vi "SwissSPAD Live_Get SS2 FPGA Parameters.vi"(6 "Live Mode":bool, 8 "Error In":errorcluster, 10 "Bifile Path":path, 11 "SS2 DAQ Parameters":T1 {"Sync Period" min=0.0 max=4.294967295; "Laser Period" min=0.0 max=4.294967295}) -> (0 "Error Out":errorcluster, 1 "#8-bit Images per Set":u32, 2 "SS2 FPGA DAQ Parameters":u32[](array[numeric]), 3 "SS2 FPGA DAQ Addresses":i32[](array[numeric]), 5 "Discard First Image":bool)   [LabVIEW 2021]
uses:
  SwissSPAD Live_SS2 DAQ Parameters 3.ctl
  SwissSPAD Live_SS2 Gate Definition.ctl
  <vilib>/Utility/error.llb/Error Cluster From Error Code.vi
  <vilib>/ErrorRing/Error Ring.xnode
panel:
  out "Buffer Size (#8-bit Images)":u32
  in  "Current Image Set":i32
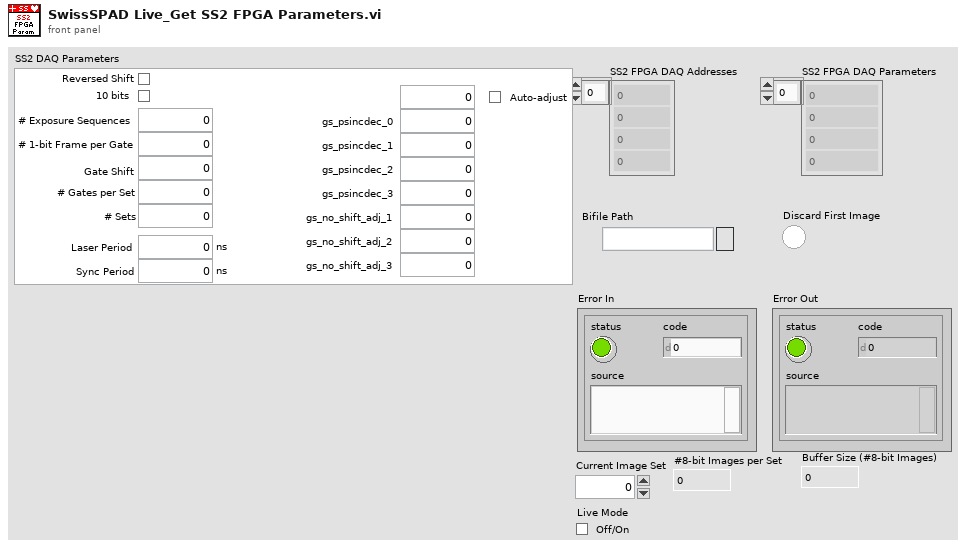
[diagram p1: front panel]
types:
  T1 = typedef "SwissSPAD Live_SS2 DAQ Parameters 3.ctl" = cluster{"10 bits":bool, "# Exposure Sequences":u32, "# 1-bit Frame per Gate":u32, "Gate Shift":u32, "# Gates per Set":u32, "# Sets":u32, "Laser Period":dbl[unit], "Sync Period":dbl[unit], "Gate Offset":u32, "Auto-adjust Gate Offset":bool, "Gate Definition":T2, "Reversed Shift":bool}
  T2 = typedef "SwissSPAD Live_SS2 Gate Definition.ctl" = cluster{"gs_psincdec_0":u32, "gs_psincdec_1":u32, "gs_psincdec_2":u32, "gs_psincdec_3":u32, "gs_no_shift_adj_1":u32, "gs_no_shift_adj_2":u32, "gs_no_shift_adj_3":u32}
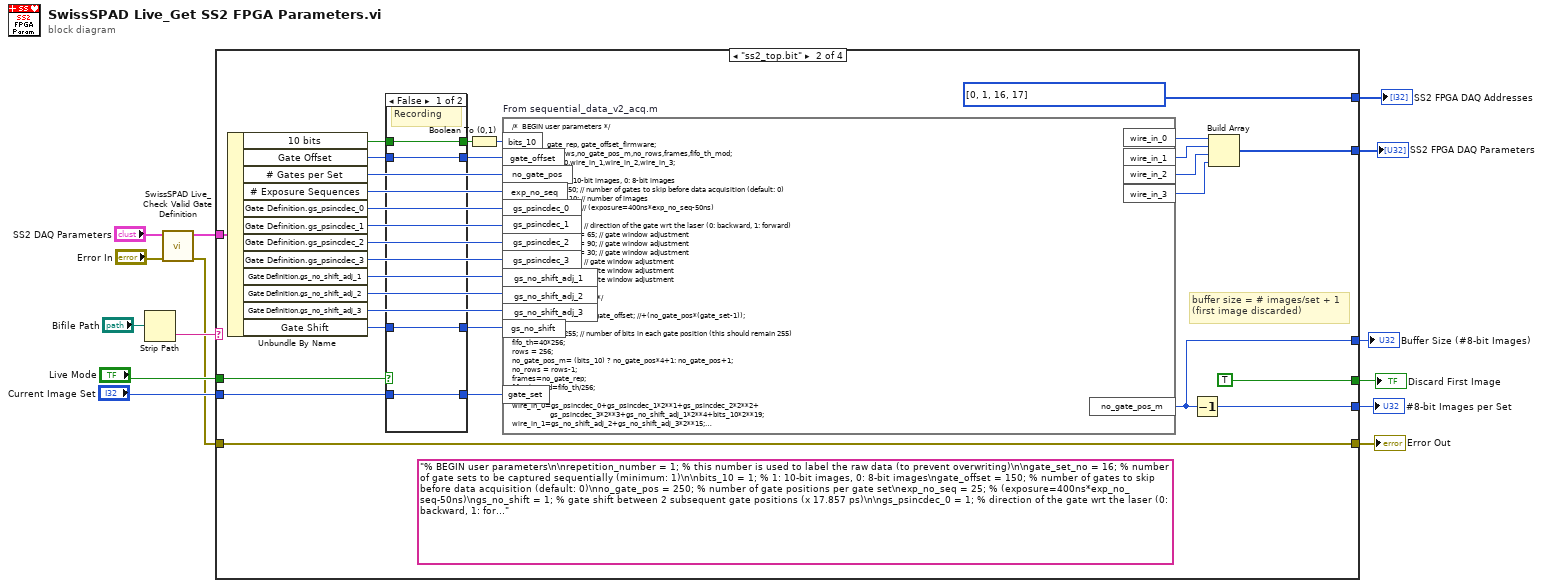
[diagram p0: block diagram]
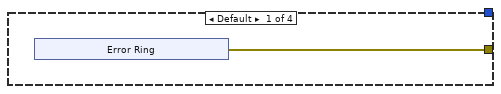
[diagram p2: hidden frame]
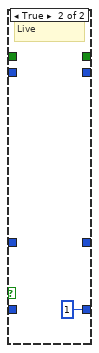
[diagram p3: hidden frame]
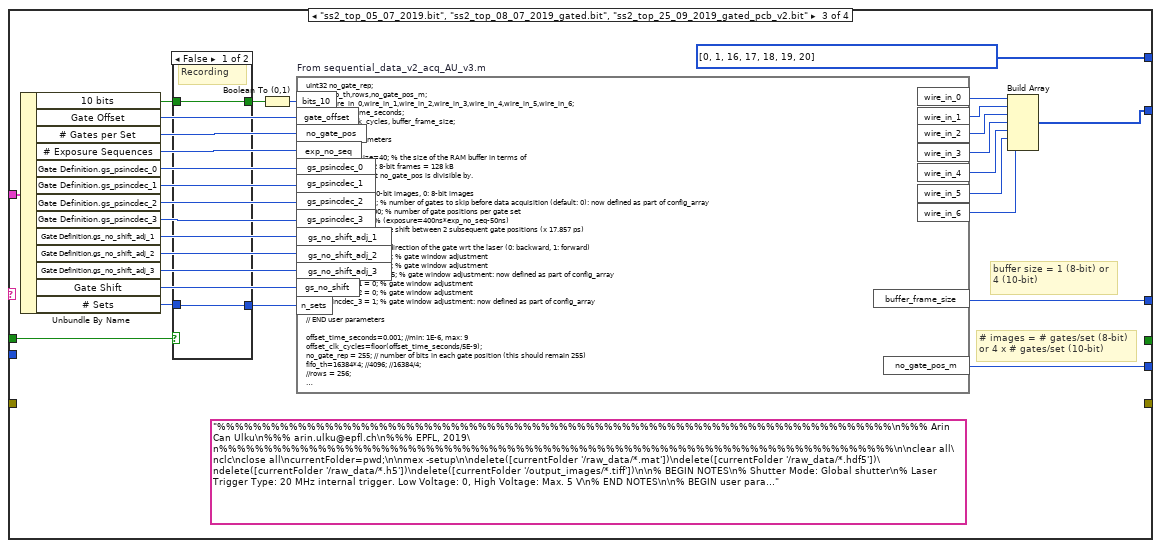
[diagram p4: hidden frame]
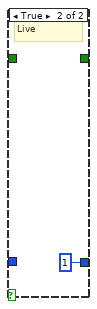
[diagram p5: hidden frame]
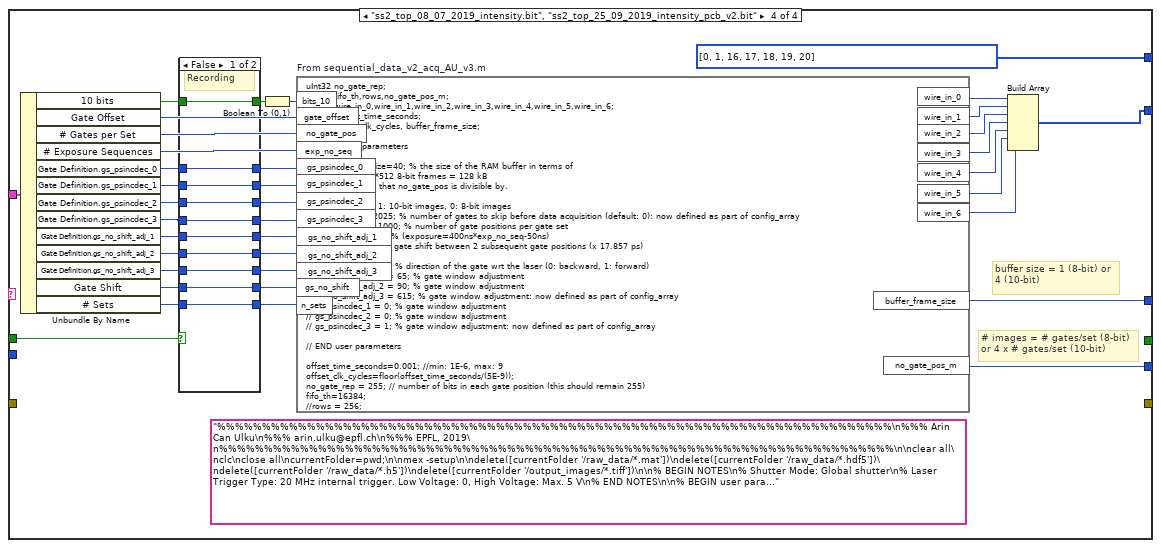
[diagram p6: hidden frame]
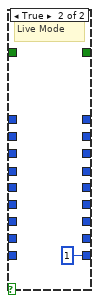
[diagram p7: hidden frame]
diagram:
  n1 = Strip Path(path="Bifile Path") -> (name=w7:string)  [unwired: 1 out]
  n2 = call "SwissSPAD Live_Check Valid Gate Definition.vi"("Error In"="Error In", "SS2 DAQ Parameters in"="SS2 DAQ Parameters") -> ("Error Out"=w4:errorcluster, "SS2 DAQ Parameters out"=w5:T1)  [unwired: 8 in]
  n3 = case shown="\"ss2_top.bit\"" w7 {
    tunnel: [_ w45 w79 w119] -> w14
    tunnel: [_ i32[] [0, 1, 16, 17] ("SS2 FPGA DAQ Addresses") i32[] [0, 1, 16, 17, 18, 19, 20] ("SS2 FPGA DAQ Addresses") i32[] [0, 1, 16, 17, 18, 19, 20] ("SS2 FPGA DAQ Addresses")] -> w13
    tunnel: w5 -> [_ w43 w77 w117]
    tunnel: "Current Image Set" -> [_ w29 _ _]
    tunnel: [_ w24 w69 w105] -> w10
    tunnel: "Live Mode" -> [_ w32 w61 w113]
    tunnel: w4 -> [_ w25 _ _]
    tunnel: [w15 w25 _ _] -> w6
    tunnel: [_ TRUE ("Discard First Image") _ _] -> w2
    tunnel: [_ w22 w56 w88] -> w1
    frame Default {
      n4 = xnode "Error Ring"() -> ("error out"=w15:errorcluster)
    }
    frame "ss2_top.bit" {
      (unwired) "% BEGIN user parameters\n\nrepetition_number = 1; % this number is used to label the raw data (to prevent overwriting)\n\ngate_set_no = 16; % number of gate sets to be captured sequentially (minimum: 1)\n\nbits_10 = 1; % 1: 10-bit images, 0: 8-bit images\ngate_offset = 150; % number of gates to skip before data acquisition (default: 0)\nno_gate_pos = 250; % number of gate positions per gate set\nexp_no_seq = 25; % (exposure=400ns*exp_no_seq-50ns)\ngs_no_shift = 1; % gate shift between 2 subsequent gate positions (x 17.857 ps)\n\ngs_psincdec_0 = 1; % direction of the gate wrt the laser (0: backward, 1: forward)\ngs_no_shift_adj_1 = 65; % gate window adjustment\ngs_no_shift_adj_2 = 90; % gate window adjustment\ngs_no_shift_adj_3 = 85; % gate window adjustment\ngs_psincdec_1 = 0; % gate window adjustment\ngs_psincdec_2 = 0; % gate window adjustment\ngs_psincdec_3 = 0; % gate window adjustment\n\n% END user parameters\n\ndisp('ACQUIRING DATA...')\n\nno_gate_rep = 255; % number of bits in each gate position (this should remain 255)\nfifo_th=40*256;\nrows = 256;\nif bits_10==1\n    no_gate_pos_m=(no_gate_pos*4)+1;\nelse\n    no_gate_pos_m=no_gate_pos+1;\nend\nno_rows = rows-1;\nframes=no_gate_rep;\ngate_set_no_str=int2str(gate_set_no);\nfifo_th_mod=fifo_th/256;\n\nCC=cell(1,gate_set_no);\n\nfor gate_set=1:gate_set_no\n\n    gate_set_str=int2str(gate_set);\n    gate_offset_firmware = gate_offset+(no_gate_pos*(gate_set-1));\n\n    setenv('MW_MINGW64_LOC','C:\\TDM-GCC-64')\n    dev = openFPGA();\n\n    %% ENTER THE BIT FILE DIRECTORY TO THE LINE BELOW %%\n    bitfile = [currentFolder '\\bit_file\\ss2_top.bit'];\n    z_status=configureFPGA(dev, bitfile);\n\n    wire_in_0=gs_psincdec_0+gs_psincdec_1*2^1+gs_psincdec_2*2^2+gs_psincdec_3*2^3+gs_no_shift_adj_1*2^4+bits_10*2^19;\n    setwireinvalue(dev,int32(hex2dec('00')),wire_in_0,wire_in_0)\n    updatewireins(dev)\n    wire_in_1=gs_no_shift_adj_2+gs_no_shift_adj_3*2^15;\n    setwireinvalue(dev,int32(hex2dec('01')),wire_in_1,wire_in_1)\n    updatewireins(dev)\n    wire_in_2=fifo_th_mod+no_gate_pos_m*2^8+gs_no_shift*2^24;\n    setwireinvalue(dev,int32(hex2dec('10')),wire_in_2,wire_in_2)\n    updatewireins(dev)\n    wire_in_3=exp_no_seq+gate_offset_firmware*2^16;\n    setwireinvalue(dev,int32(hex2dec('11')),wire_in_3,wire_in_3)\n    updatewireins(dev)\n\n    % BEGIN SAVE\n\n    activatetriggerin(dev,int32(hex2dec('40')),0)\n    activatetriggerin(dev,int32(hex2dec('40')),1)\n\n    disp(['GATE SET:' gate_set_str '/' gate_set_no_str ' --- ACQUIRING DATA...'])\n    tic\n    CC{gate_set}=readfromblockpipeout(dev,int32(hex2dec('A0')),16*256*4,(512*256)*no_gate_pos_m);\n    toc\n    \n    closeFPGA(dev);"
      # "buffer size = # images/set + 1\n(first image discarded)"
      n5 = Unbundle By Name(w43) -> ("10 bits"=w31:bool, "Gate Offset"=w21:u32, "# Gates per Set"=w41:u32, "# Exposure Sequences"=w40:u32, "Gate Definition.gs_psincdec_0"=w39:u32, "Gate Definition.gs_psincdec_1"=w38:u32, "Gate Definition.gs_psincdec_2"=w37:u32, "Gate Definition.gs_psincdec_3"=w36:u32, "Gate Definition.gs_no_shift_adj_1"=w35:u32, "Gate Definition.gs_no_shift_adj_2"=w34:u32, "Gate Definition.gs_no_shift_adj_3"=w33:u32, "Gate Shift"=w27:u32)
      n6 = case shown="False" w32 {
        tunnel: w31 -> [w53 _]
        tunnel: [w53 _] -> w30
        tunnel: w29 -> [w52 _]
        tunnel: [w52 1 ("Current Image Set")] -> w28
        tunnel: w27 -> [w51 _]
        tunnel: [w51 _] -> w26
        tunnel: w21 -> [w50 _]
        tunnel: [w50 _] -> w20
        frame False {
          # "Recording"
        }
        frame True {
          # "Live"
        }
      }
      n7 = Boolean To (0,1)(Boolean=w30) -> (0, 1=w42:i16)
      n8 = formula code="/*  BEGIN user parameters */\n\nuInt32 no_gate_rep, gate_offset_firmware;\nuInt32 fifo_th,rows,no_gate_pos_m,no_rows,frames,fifo_th_mod;\nuInt32 wire_in_0,wire_in_1,wire_in_2,wire_in_3;\n\n//bits_10 = 0; // 1: 10-bit images, 0: 8-bit images\n//gate_offset = 650; // number of gates to skip before data acquisition (default: 0)\n//no_gate_pos = 10; // number of images\n//exp_no_seq = 100; // (exposure=400ns*exp_no_seq-50ns)\n\n//gs_psincdec_0 = 1; // direction of the gate wrt the laser (0: backward, 1: forward)\n//gs_no_shift_adj_1 = 65; // gate window adjustment\n//gs_no_shift_adj_2 = 90; // gate window adjustment\n//gs_no_shift_adj_3 = 30; // gate window adjustment\n//gs_psincdec_1 = 0; // gate window adjustment\n//gs_psincdec_2 = 0; // gate window adjustment\n//gs_psincdec_3 = 0; // gate window adjustment\n\n/*  END user parameters */\n\ngate_offset_firmware = gate_offset; //+(no_gate_pos*(gate_set-1));\n\nno_gate_rep = 255; // number of bits in each gate position (this should remain 255)\nfifo_th=40*256;\nrows = 256;\nno_gate_pos_m= (bits_10) ? no_gate_pos*4+1: no_gate_pos+1;\nno_rows = rows-1;\nframes=no_gate_rep;\nfifo_th_mod=fifo_th/256;\n\nwire_in_0=gs_psincdec_0+gs_psincdec_1*2**1+gs_psincdec_2*2**2+\n                   gs_psincdec_3*2**3+gs_no_shift_adj_1*2**4+bits_10*2**19;\nwire_in_1=gs_no_shift_adj_2+gs_no_shift_adj_3*2**15;\nwire_in_2=fifo_th_mod+no_gate_pos_m*2**8+gs_no_shift*2**24;\nwire_in_3=exp_no_seq+gate_offset_firmware*2**16;" "From sequential_data_v2_acq.m"("bits_10"=w42, "gate_offset"=w20, "no_gate_pos"=w41, "exp_no_seq"=w40, "gs_psincdec_0"=w39, "gs_psincdec_1"=w38, "gs_psincdec_2"=w37, "gs_psincdec_3"=w36, "gs_no_shift_adj_1"=w35, "gs_no_shift_adj_2"=w34, "gs_no_shift_adj_3"=w33, "gate_set"=w28, "gs_no_shift"=w26) -> ("wire_in_1"=w48:u32, "wire_in_0"=w49:u32, "wire_in_2"=w47:u32, "wire_in_3"=w46:u32, "no_gate_pos_m"=w22:u32)
      n9 = Decrement(x=w22) -> (x-1=w24:u32)
      n10 = Build Array(w49, w48, w47, w46) -> (w45:u32[])
    }
    frame "ss2_top_05_07_2019.bit", "ss2_top_08_07_2019_gated.bit", "ss2_top_25_09_2019_gated_pcb_v2.bit" {
      (unwired) "%%%%%%%%%%%%%%%%%%%%%%%%%%%%%%%%%%%%%%%%%%%%%%%%%%%%%%%%%%%%%%%%%%%%%%%%%%%\n%%% Arin Can Ulku\n%%% arin.ulku@epfl.ch\n%%% EPFL, 2019\n%%%%%%%%%%%%%%%%%%%%%%%%%%%%%%%%%%%%%%%%%%%%%%%%%%%%%%%%%%%%%%%%%%%%%%%%%%%\n\nclear all\nclc\nclose all\ncurrentFolder=pwd;\n\nmex -setup\n\ndelete([currentFolder '/raw_data/*.mat'])\ndelete([currentFolder '/raw_data/*.hdf5'])\ndelete([currentFolder '/raw_data/*.h5'])\ndelete([currentFolder '/output_images/*.tiff'])\n\n% BEGIN NOTES\n% Shutter Mode: Global shutter\n% Laser Trigger Type: 20 MHz internal trigger. Low Voltage: 0, High Voltage: Max. 5 V\n% END NOTES\n\n% BEGIN user parameters\n\n%%%%%%%%%%%%%%%%%%%%%%%%%%%%%%%%%%%%%%%%%%%%%%%%%%%%%\n% Added by XM for hdf5 saving and automation purposes\n\nfile_root_name = 'DCR study'; % root file name\nrepetition_number = 1;                 % number of repetitions per config\nrepetition_number_str = int2str(repetition_number);\nconfig_choice = [3];                 % define which config(s) to use\n% For all config, use [1 2 3 4 5 6 7]\n% For a single config, e.g. 3, use [3]\nconfig_number = length(config_choice);\n\n% Don't modify the array below unless you know what you are doing...\nconfig_array = struct('gate_offset', {2690,2640,2570,2430,2300,2170,2025},...\n    'gs_no_shift_adj_3',{85,30,55,195,335,475,615},...\n    'gs_psincdec_3',{0,0,1,1,1,1,1},...\n    'gate_width_ns',{10.8,11.7,13.1,15.5,17.9,20.3,22.8});\n% offset array for Arin's series: {2690,2640,2570,2430,2300,2170,2025}\nfile_version = 'SS2 0.1';               % do not modify\nsoftware_name = 'sequential_data_v2_acq.m'; % do not modify\nsoftware_version = '64-bit';            % do not modify\nfirmware_name = 'ss2_top_05_07_2019.bit';          % do not modify\nfirmware_version = '07-05-2019';        % modify when firmware has been updated\nsample_description = 'DCR Study as a function of integration time'; % user-defined\nauthor = 'X. Michalet';                 % user-defined\nlaser_f_MHz = 20;                       % do not modify\npixel_x = 512;                          % do not modify\npixel_y = 256;                          % do not modify\ngate_step_ps = 17.857;                  % do not modify, might change if firmware changes\n\n% end XM additions\n%%%%%%%%%%%%%%%%%%%%%%%%%%%%%%%%%%%%%%\n\nbuffer_frame_size=40; % the size of the RAM buffer in terms of equivalent 256*512 frames\n% choose a value that no_gate_pos is divisible by.\n\nbits_10 = 0; % 1: 10-bit images, 0: 8-bit images\n%gate_offset = 2025; % number of gates to skip before data acquisition (default: 0): now defined as part of config_array\nno_gate_pos = 1000; % number of gate positions per gate set\nexp_no_seq = 25; % (exposure=400ns*exp_no_seq-50ns)\ngs_no_shift = 1; % gate shift between 2 subsequent gate positions (x 17.857 ps)\n\ngs_psincdec_0 = 1; % direction of the gate wrt the laser (0: backward, 1: forward)\ngs_no_shift_adj_1 = 65; % gate window adjustment\ngs_no_shift_adj_2 = 90; % gate window adjustment\n%gs_no_shift_adj_3 = 615; % gate window adjustment: now defined as part of config_array\ngs_psincdec_1 = 0; % gate window adjustment\ngs_psincdec_2 = 0; % gate window adjustment\n%gs_psincdec_3 = 1; % gate window adjustment: now defined as part of config_array\n\n% END user parameters\n\ngate_set_no = 1; % number of gate sets to be captured sequentially (minimum: 1)\noffset_time_seconds=0.001; %% min: 1E-6, max: 9\noffset_clk_cycles=floor(offset_time_seconds/(5E-9));\nno_gate_rep = 255; % number of bits in each gate position (this should remain 255)\nfifo_th=16384/4;\nrows = 256;\nif bits_10==1\n    no_gate_pos_m=(no_gate_pos*4);\nelse\n    no_gate_pos_m=no_gate_pos;\nend\nno_rows = rows-1;\nframes=no_gate_rep;\n\nsetenv('MW_MINGW64_LOC','C:\\TDM-GCC-64')\ndev = openFPGA();\nbitfile = [currentFolder '\\bit_file\\ss2_top_08_07_2019_intensity.bit'];\nz_status=configureFPGA(dev, bitfile);\n\nfor j=1:config_number\n    config = config_choice(j);\n    gate_offset = config_array(config).gate_offset;\n    gs_no_shift_adj_3 = config_array(config).gs_no_shift_adj_3;\n    gs_psincdec_3 = config_array(config).gs_psincdec_3;\n    gate_width_ns = config_array(config).gate_width_ns;\n    config_number_str = [' (config ' int2str(config) ')'];\n    file_name = [file_root_name config_number_str];\n    \n    %%%%%%%%%%%%%%%%%%%%%%%%%%%%%%%%%%%%%%\n    % Added by XM for hdf5 saving purposes\n\n    hdf5write([currentFolder '\\raw_data\\' file_name '.hdf5'],'/SS2_file_version',file_version);\n    hdf5write([currentFolder '\\raw_data\\' file_name '.hdf5'],'/daq_parameters/pixel_x',pixel_x,'WriteMode', 'append');\n    hdf5write([currentFolder '\\raw_data\\' file_name '.hdf5'],'/daq_parameters/pixel_y',pixel_y,'WriteMode', 'append');\n    hdf5write([currentFolder '\\raw_data\\' file_name '.hdf5'],'/daq_parameters/gate_set_no',gate_set_no,'WriteMode', 'append');\n    hdf5write([currentFolder '\\raw_data\\' file_name '.hdf5'],'/daq_parameters/bits_10',bits_10,'WriteMode', 'append');\n    hdf5write([currentFolder '\\raw_data\\' file_name '.hdf5'],'/daq_parameters/gate_offset',gate_offset,'WriteMode', 'append');\n    hdf5write([currentFolder '\\raw_data\\' file_name '.hdf5'],'/daq_parameters/no_gate_pos',no_gate_pos,'WriteMode', 'append');\n    hdf5write([currentFolder '\\raw_data\\' file_name '.hdf5'],'/daq_parameters/exp_no_seq',exp_no_seq,'WriteMode', 'append');\n    hdf5write([currentFolder '\\raw_data\\' file_name '.hdf5'],'/daq_parameters/gs_no_shift',gs_no_shift,'WriteMode', 'append');\n    hdf5write([currentFolder '\\raw_data\\' file_name '.hdf5'],'/daq_parameters/gs_psincdec_0',gs_psincdec_0,'WriteMode', 'append');\n    hdf5write([currentFolder '\\raw_data\\' file_name '.hdf5'],'/daq_parameters/gs_no_shift_adj_1',gs_no_shift_adj_1,'WriteMode', 'append');\n    hdf5write([currentFolder '\\raw_data\\' file_name '.hdf5'],'/daq_parameters/gs_no_shift_adj_2',gs_no_shift_adj_2,'WriteMode', 'append');\n    hdf5write([currentFolder '\\raw_data\\' file_name '.hdf5'],'/daq_parameters/gs_no_shift_adj_3',gs_no_shift_adj_3,'WriteMode', 'append');\n    hdf5write([currentFolder '\\raw_data\\' file_name '.hdf5'],'/daq_parameters/gs_psincdec_1',gs_psincdec_1,'WriteMode', 'append');\n    hdf5write([currentFolder '\\raw_data\\' file_name '.hdf5'],'/daq_parameters/gs_psincdec_2',gs_psincdec_2,'WriteMode', 'append');\n    hdf5write([currentFolder '\\raw_data\\' file_name '.hdf5'],'/daq_parameters/gs_psincdec_3',gs_psincdec_3,'WriteMode', 'append');\n    hdf5write([currentFolder '\\raw_data\\' file_name '.hdf5'],'/daq_parameters/gate_step_ps',gate_step_ps,'WriteMode', 'append');\n    hdf5write([currentFolder '\\raw_data\\' file_name '.hdf5'],'/daq_parameters/gate_width_ns',gate_width_ns,'WriteMode', 'append');\n    hdf5write([currentFolder '\\raw_data\\' file_name '.hdf5'],'/daq_parameters/shutter_mode','global shutter','WriteMode', 'append');\n    hdf5write([currentFolder '\\raw_data\\' file_name '.hdf5'],'/daq_parameters/laser_f_MHz',laser_f_MHz,'WriteMode', 'append');\n\n    hdf5write([currentFolder '\\raw_data\\' file_name '.hdf5'],'/data_information/description',[sample_description config_number_str],'WriteMode', 'append');\n    hdf5write([currentFolder '\\raw_data\\' file_name '.hdf5'],'/data_information/author',author,'WriteMode', 'append');\n    hdf5write([currentFolder '\\raw_data\\' file_name '.hdf5'],'/data_information/software_name',software_name,'WriteMode', 'append');\n    hdf5write([currentFolder '\\raw_data\\' file_name '.hdf5'],'/data_information/software_version',software_version,'WriteMode', 'append');\n    hdf5write([currentFolder '\\raw_data\\' file_name '.hdf5'],'/data_information/firmware_name',firmware_name,'WriteMode', 'append');\n    hdf5write([currentFolder '\\raw_data\\' file_name '.hdf5'],'/data_information/firmware_version',firmware_version,'WriteMode', 'append');\n\n\n    for i=1:repetition_number\n%         exp_no_seq = 10*i;\n        repetition_number_str = [' exp = ' int2str(exp_no_seq)];       \n\n        wire_in_0=gs_psincdec_0+gs_psincdec_1*2^1+gs_psincdec_2*2^2+gs_psincdec_3*2^3+gs_no_shift_adj_1*2^4+bits_10*2^19;\n        setwireinvalue(dev,int32(hex2dec('00')),wire_in_0,wire_in_0)\n        updatewireins(dev)\n        wire_in_1=gs_no_shift_adj_2+gs_no_shift_adj_3*2^15;\n        setwireinvalue(dev,int32(hex2dec('01')),wire_in_1,wire_in_1)\n        updatewireins(dev)\n        wire_in_2=no_gate_pos_m*2^8;\n        setwireinvalue(dev,int32(hex2dec('10')),wire_in_2,wire_in_2)\n        updatewireins(dev)\n        wire_in_3=exp_no_seq+gate_offset*2^16;\n        setwireinvalue(dev,int32(hex2dec('11')),wire_in_3,wire_in_3)\n        updatewireins(dev)\n        wire_in_4=gs_no_shift;\n        setwireinvalue(dev,int32(hex2dec('12')),wire_in_4,wire_in_4)\n        updatewireins(dev)\n        wire_in_5=fifo_th;\n        setwireinvalue(dev,int32(hex2dec('13')),wire_in_5,wire_in_5)\n        updatewireins(dev)\n        wire_in_6=offset_clk_cycles;\n        setwireinvalue(dev,int32(hex2dec('14')),wire_in_6,wire_in_6)\n        updatewireins(dev)\n\n        % BEGIN SAVE\n\n        rep_no=fix(no_gate_pos_m/buffer_frame_size);\n        [daq_time]=ss2_daq_hdf5_v3(file_name,rep_no,dev,int32(hex2dec('A0')),16384,(512*256)*buffer_frame_size);\n    \n        %%%%%%%%%%%%%%%%%%%%%%%%%%%%%%%%%%%%%%\n        % Added by XM for hdf5 saving purposes\n\n        disp(['Elapsed DAQ time: ' num2str(daq_time) ' sec']);\n\n        % end XM additions\n        %%%%%%%%%%%%%%%%%%%%%%%%%%%%%%%%%%%%%%\n\n%         updatewireouts(dev);\n%         fsm_state = dec2hex(getwireoutvalue(dev,int32(hex2dec('20'))));    \n        updatewireouts(dev);\n        fsm_state_2 = dec2hex(getwireoutvalue(dev,int32(hex2dec('21'))));\n\n        beep\n \n        disp([10 'ACQUISITION COMPLETED. YOU CAN TURN OFF THE LASER NOW.' 10])\n%         fsm_state_int=str2double(fsm_state_2);\n%         if fsm_state_int==2\n%             disp(['USB DATA TRANSFER SUCCESSFUL!' 10])\n%         else\n%             disp(['USB DATA TRANSFER FAILED!' 10])\n%         end\n        \n%         file_number_str=int2str(i);\n%         disp(['SAVING HDF5 RAW DATA... File ' file_number_str ' of ' repetition_number_str config_number_str 10])\n\n    end\nend\n\ncloseFPGA(dev);\n\nhdf5write([currentFolder '\\raw_data\\' file_name '.hdf5'],'/daq_time_s',daq_time,'WriteMode', 'append');\n\n% end XM additions\n%%%%%%%%%%%%%%%%%%%%%%%%%%%%%%%%%%%%%%\n    \n%% \n\n%%%%%%%%%%%%%%%%%%%%%%%%%%%%%%%%%%%%%%\n% Added by AU for testing purposes\n\n% disp([10 'SAVING .MAT RAW DATA...' 10])\n% \n% tic\n% \n% save([currentFolder '\\raw_data\\raw_data_1.mat'],'SS2_DATA', '-v7.3');\n% \n% toc\n\n% end AU additions\n%%%%%%%%%%%%%%%%%%%%%%%%%%%%%%%%%%%%%%\n\ndisp([10 'DONE.'])\n\n%disp('SAVING MATLAB RAW DATA...')\n\n%tic\n%save([currentFolder '\\raw_data\\' file_name '_' file_number_str '.mat'],'CC');\n%toc\n\nbeep"
      # "# images = # gates/set (8-bit)\nor 4 x # gates/set (10-bit)"
      # "buffer size = 1 (8-bit) or 4 (10-bit)"
      n11 = Unbundle By Name(w77) -> ("10 bits"=w60:bool, "Gate Offset"=w55:u32, "# Gates per Set"=w75:u32, "# Exposure Sequences"=w74:u32, "Gate Definition.gs_psincdec_0"=w68:u32, "Gate Definition.gs_psincdec_1"=w67:u32, "Gate Definition.gs_psincdec_2"=w66:u32, "Gate Definition.gs_psincdec_3"=w65:u32, "Gate Definition.gs_no_shift_adj_1"=w64:u32, "Gate Definition.gs_no_shift_adj_2"=w63:u32, "Gate Definition.gs_no_shift_adj_3"=w62:u32, "Gate Shift"=w73:u32, "# Sets"=w58:u32)
      n12 = case shown="False" w61 {
        tunnel: w60 -> [w85 _]
        tunnel: [w85 _] -> w59
        tunnel: w58 -> [w84 _]
        tunnel: [w84 u32 1 ("# Sets")] -> w57
        frame False {
          # "Recording"
        }
        frame True {
          # "Live"
        }
      }
      n13 = Boolean To (0,1)(Boolean=w59) -> (0, 1=w76:i16)
      n14 = formula code="uInt32 no_gate_rep;\nuInt32 fifo_th,rows,no_gate_pos_m;\nuInt32 wire_in_0,wire_in_1,wire_in_2,wire_in_3,wire_in_4,wire_in_5,wire_in_6;\nfloat64 offset_time_seconds;\nuInt32 offset_clk_cycles, buffer_frame_size;\n\n// BEGIN user parameters\n\n// buffer_frame_size=40; % the size of the RAM buffer in terms of \n// equivalent 256*512 8-bit frames = 128 kB\n// choose a value that no_gate_pos is divisible by.\n\n// bits_10 = 0; % 1: 10-bit images, 0: 8-bit images\n// gate_offset = 2025; % number of gates to skip before data acquisition (default: 0): now defined as part of config_array\n// no_gate_pos = 1000; % number of gate positions per gate set\n// exp_no_seq = 25; % (exposure=400ns*exp_no_seq-50ns)\n// gs_no_shift = 1; % gate shift between 2 subsequent gate positions (x 17.857 ps)\n\n// gs_psincdec_0 = 1; % direction of the gate wrt the laser (0: backward, 1: forward)\n// gs_no_shift_adj_1 = 65; % gate window adjustment\n// gs_no_shift_adj_2 = 90; % gate window adjustment\n// gs_no_shift_adj_3 = 615; % gate window adjustment: now defined as part of config_array\n// gs_psincdec_1 = 0; % gate window adjustment\n// gs_psincdec_2 = 0; % gate window adjustment\n// gs_psincdec_3 = 1; % gate window adjustment: now defined as part of config_array\n\n// END user parameters\n\noffset_time_seconds=0.001; //min: 1E-6, max: 9\noffset_clk_cycles=floor(offset_time_seconds/5E-9);\nno_gate_rep = 255; // number of bits in each gate position (this should remain 255)\nfifo_th=16384*4; //4096; //16384/4;\n//rows = 256;\n\n no_gate_pos_m = (bits_10 ==1) ? no_gate_pos*4 : no_gate_pos;\nbuffer_frame_size = (bits_10 ==1) ? 4 : 1;\n//= no_gate_pos_m; // e.g. bits_10 = 1, no_gate_pos = 100 >> buffer = 50 MB\n//no_gate_pos_m *= n_sets; \n\n//no_rows = rows-1;\n//frames=no_gate_rep;\n\nwire_in_0=gs_psincdec_0+gs_psincdec_1*2**1+gs_psincdec_2*2**2+gs_psincdec_3*2**3+gs_no_shift_adj_1*2**4+bits_10*2**19;\nwire_in_1=gs_no_shift_adj_2+gs_no_shift_adj_3*2**15;\nwire_in_2=no_gate_pos_m*2**8;\nwire_in_3=exp_no_seq+gate_offset*2**16;\nwire_in_4=gs_no_shift;\nwire_in_5=fifo_th;\nwire_in_6=offset_clk_cycles;" "From sequential_data_v2_acq_AU_v3.m"("bits_10"=w76, "gate_offset"=w55, "no_gate_pos"=w75, "exp_no_seq"=w74, "gs_psincdec_0"=w68, "gs_psincdec_1"=w67, "gs_psincdec_2"=w66, "gs_psincdec_3"=w65, "gs_no_shift_adj_1"=w64, "gs_no_shift_adj_2"=w63, "gs_no_shift_adj_3"=w62, "gs_no_shift"=w73, "n_sets"=w57) -> ("wire_in_1"=w82:u32, "wire_in_0"=w83:u32, "wire_in_2"=w81:u32, "wire_in_3"=w80:u32, "no_gate_pos_m"=w69:u32, "wire_in_4"=w72:u32, "wire_in_5"=w71:u32, "wire_in_6"=w70:u32, "buffer_frame_size"=w56:u32)
      n15 = Build Array(w83, w82, w81, w80, w72, w71, w70) -> (w79:u32[])
    }
    frame "ss2_top_08_07_2019_intensity.bit", "ss2_top_25_09_2019_intensity_pcb_v2.bit" {
      (unwired) "%%%%%%%%%%%%%%%%%%%%%%%%%%%%%%%%%%%%%%%%%%%%%%%%%%%%%%%%%%%%%%%%%%%%%%%%%%%\n%%% Arin Can Ulku\n%%% arin.ulku@epfl.ch\n%%% EPFL, 2019\n%%%%%%%%%%%%%%%%%%%%%%%%%%%%%%%%%%%%%%%%%%%%%%%%%%%%%%%%%%%%%%%%%%%%%%%%%%%\n\nclear all\nclc\nclose all\ncurrentFolder=pwd;\n\nmex -setup\n\ndelete([currentFolder '/raw_data/*.mat'])\ndelete([currentFolder '/raw_data/*.hdf5'])\ndelete([currentFolder '/raw_data/*.h5'])\ndelete([currentFolder '/output_images/*.tiff'])\n\n% BEGIN NOTES\n% Shutter Mode: Global shutter\n% Laser Trigger Type: 20 MHz internal trigger. Low Voltage: 0, High Voltage: Max. 5 V\n% END NOTES\n\n% BEGIN user parameters\n\n%%%%%%%%%%%%%%%%%%%%%%%%%%%%%%%%%%%%%%%%%%%%%%%%%%%%%\n% Added by XM for hdf5 saving and automation purposes\n\nfile_root_name = 'DCR study'; % root file name\nrepetition_number = 1;                 % number of repetitions per config\nrepetition_number_str = int2str(repetition_number);\nconfig_choice = [3];                 % define which config(s) to use\n% For all config, use [1 2 3 4 5 6 7]\n% For a single config, e.g. 3, use [3]\nconfig_number = length(config_choice);\n\n% Don't modify the array below unless you know what you are doing...\nconfig_array = struct('gate_offset', {2690,2640,2570,2430,2300,2170,2025},...\n    'gs_no_shift_adj_3',{85,30,55,195,335,475,615},...\n    'gs_psincdec_3',{0,0,1,1,1,1,1},...\n    'gate_width_ns',{10.8,11.7,13.1,15.5,17.9,20.3,22.8});\n% offset array for Arin's series: {2690,2640,2570,2430,2300,2170,2025}\nfile_version = 'SS2 0.1';               % do not modify\nsoftware_name = 'sequential_data_v2_acq.m'; % do not modify\nsoftware_version = '64-bit';            % do not modify\nfirmware_name = 'ss2_top_05_07_2019.bit';          % do not modify\nfirmware_version = '07-05-2019';        % modify when firmware has been updated\nsample_description = 'DCR Study as a function of integration time'; % user-defined\nauthor = 'X. Michalet';                 % user-defined\nlaser_f_MHz = 20;                       % do not modify\npixel_x = 512;                          % do not modify\npixel_y = 256;                          % do not modify\ngate_step_ps = 17.857;                  % do not modify, might change if firmware changes\n\n% end XM additions\n%%%%%%%%%%%%%%%%%%%%%%%%%%%%%%%%%%%%%%\n\nbuffer_frame_size=40; % the size of the RAM buffer in terms of equivalent 256*512 frames\n% choose a value that no_gate_pos is divisible by.\n\nbits_10 = 0; % 1: 10-bit images, 0: 8-bit images\n%gate_offset = 2025; % number of gates to skip before data acquisition (default: 0): now defined as part of config_array\nno_gate_pos = 1000; % number of gate positions per gate set\nexp_no_seq = 25; % (exposure=400ns*exp_no_seq-50ns)\ngs_no_shift = 1; % gate shift between 2 subsequent gate positions (x 17.857 ps)\n\ngs_psincdec_0 = 1; % direction of the gate wrt the laser (0: backward, 1: forward)\ngs_no_shift_adj_1 = 65; % gate window adjustment\ngs_no_shift_adj_2 = 90; % gate window adjustment\n%gs_no_shift_adj_3 = 615; % gate window adjustment: now defined as part of config_array\ngs_psincdec_1 = 0; % gate window adjustment\ngs_psincdec_2 = 0; % gate window adjustment\n%gs_psincdec_3 = 1; % gate window adjustment: now defined as part of config_array\n\n% END user parameters\n\ngate_set_no = 1; % number of gate sets to be captured sequentially (minimum: 1)\noffset_time_seconds=0.001; %% min: 1E-6, max: 9\noffset_clk_cycles=floor(offset_time_seconds/(5E-9));\nno_gate_rep = 255; % number of bits in each gate position (this should remain 255)\nfifo_th=16384/4;\nrows = 256;\nif bits_10==1\n    no_gate_pos_m=(no_gate_pos*4);\nelse\n    no_gate_pos_m=no_gate_pos;\nend\nno_rows = rows-1;\nframes=no_gate_rep;\n\nsetenv('MW_MINGW64_LOC','C:\\TDM-GCC-64')\ndev = openFPGA();\nbitfile = [currentFolder '\\bit_file\\ss2_top_08_07_2019_intensity.bit'];\nz_status=configureFPGA(dev, bitfile);\n\nfor j=1:config_number\n    config = config_choice(j);\n    gate_offset = config_array(config).gate_offset;\n    gs_no_shift_adj_3 = config_array(config).gs_no_shift_adj_3;\n    gs_psincdec_3 = config_array(config).gs_psincdec_3;\n    gate_width_ns = config_array(config).gate_width_ns;\n    config_number_str = [' (config ' int2str(config) ')'];\n    file_name = [file_root_name config_number_str];\n    \n    %%%%%%%%%%%%%%%%%%%%%%%%%%%%%%%%%%%%%%\n    % Added by XM for hdf5 saving purposes\n\n    hdf5write([currentFolder '\\raw_data\\' file_name '.hdf5'],'/SS2_file_version',file_version);\n    hdf5write([currentFolder '\\raw_data\\' file_name '.hdf5'],'/daq_parameters/pixel_x',pixel_x,'WriteMode', 'append');\n    hdf5write([currentFolder '\\raw_data\\' file_name '.hdf5'],'/daq_parameters/pixel_y',pixel_y,'WriteMode', 'append');\n    hdf5write([currentFolder '\\raw_data\\' file_name '.hdf5'],'/daq_parameters/gate_set_no',gate_set_no,'WriteMode', 'append');\n    hdf5write([currentFolder '\\raw_data\\' file_name '.hdf5'],'/daq_parameters/bits_10',bits_10,'WriteMode', 'append');\n    hdf5write([currentFolder '\\raw_data\\' file_name '.hdf5'],'/daq_parameters/gate_offset',gate_offset,'WriteMode', 'append');\n    hdf5write([currentFolder '\\raw_data\\' file_name '.hdf5'],'/daq_parameters/no_gate_pos',no_gate_pos,'WriteMode', 'append');\n    hdf5write([currentFolder '\\raw_data\\' file_name '.hdf5'],'/daq_parameters/exp_no_seq',exp_no_seq,'WriteMode', 'append');\n    hdf5write([currentFolder '\\raw_data\\' file_name '.hdf5'],'/daq_parameters/gs_no_shift',gs_no_shift,'WriteMode', 'append');\n    hdf5write([currentFolder '\\raw_data\\' file_name '.hdf5'],'/daq_parameters/gs_psincdec_0',gs_psincdec_0,'WriteMode', 'append');\n    hdf5write([currentFolder '\\raw_data\\' file_name '.hdf5'],'/daq_parameters/gs_no_shift_adj_1',gs_no_shift_adj_1,'WriteMode', 'append');\n    hdf5write([currentFolder '\\raw_data\\' file_name '.hdf5'],'/daq_parameters/gs_no_shift_adj_2',gs_no_shift_adj_2,'WriteMode', 'append');\n    hdf5write([currentFolder '\\raw_data\\' file_name '.hdf5'],'/daq_parameters/gs_no_shift_adj_3',gs_no_shift_adj_3,'WriteMode', 'append');\n    hdf5write([currentFolder '\\raw_data\\' file_name '.hdf5'],'/daq_parameters/gs_psincdec_1',gs_psincdec_1,'WriteMode', 'append');\n    hdf5write([currentFolder '\\raw_data\\' file_name '.hdf5'],'/daq_parameters/gs_psincdec_2',gs_psincdec_2,'WriteMode', 'append');\n    hdf5write([currentFolder '\\raw_data\\' file_name '.hdf5'],'/daq_parameters/gs_psincdec_3',gs_psincdec_3,'WriteMode', 'append');\n    hdf5write([currentFolder '\\raw_data\\' file_name '.hdf5'],'/daq_parameters/gate_step_ps',gate_step_ps,'WriteMode', 'append');\n    hdf5write([currentFolder '\\raw_data\\' file_name '.hdf5'],'/daq_parameters/gate_width_ns',gate_width_ns,'WriteMode', 'append');\n    hdf5write([currentFolder '\\raw_data\\' file_name '.hdf5'],'/daq_parameters/shutter_mode','global shutter','WriteMode', 'append');\n    hdf5write([currentFolder '\\raw_data\\' file_name '.hdf5'],'/daq_parameters/laser_f_MHz',laser_f_MHz,'WriteMode', 'append');\n\n    hdf5write([currentFolder '\\raw_data\\' file_name '.hdf5'],'/data_information/description',[sample_description config_number_str],'WriteMode', 'append');\n    hdf5write([currentFolder '\\raw_data\\' file_name '.hdf5'],'/data_information/author',author,'WriteMode', 'append');\n    hdf5write([currentFolder '\\raw_data\\' file_name '.hdf5'],'/data_information/software_name',software_name,'WriteMode', 'append');\n    hdf5write([currentFolder '\\raw_data\\' file_name '.hdf5'],'/data_information/software_version',software_version,'WriteMode', 'append');\n    hdf5write([currentFolder '\\raw_data\\' file_name '.hdf5'],'/data_information/firmware_name',firmware_name,'WriteMode', 'append');\n    hdf5write([currentFolder '\\raw_data\\' file_name '.hdf5'],'/data_information/firmware_version',firmware_version,'WriteMode', 'append');\n\n\n    for i=1:repetition_number\n%         exp_no_seq = 10*i;\n        repetition_number_str = [' exp = ' int2str(exp_no_seq)];       \n\n        wire_in_0=gs_psincdec_0+gs_psincdec_1*2^1+gs_psincdec_2*2^2+gs_psincdec_3*2^3+gs_no_shift_adj_1*2^4+bits_10*2^19;\n        setwireinvalue(dev,int32(hex2dec('00')),wire_in_0,wire_in_0)\n        updatewireins(dev)\n        wire_in_1=gs_no_shift_adj_2+gs_no_shift_adj_3*2^15;\n        setwireinvalue(dev,int32(hex2dec('01')),wire_in_1,wire_in_1)\n        updatewireins(dev)\n        wire_in_2=no_gate_pos_m*2^8;\n        setwireinvalue(dev,int32(hex2dec('10')),wire_in_2,wire_in_2)\n        updatewireins(dev)\n        wire_in_3=exp_no_seq+gate_offset*2^16;\n        setwireinvalue(dev,int32(hex2dec('11')),wire_in_3,wire_in_3)\n        updatewireins(dev)\n        wire_in_4=gs_no_shift;\n        setwireinvalue(dev,int32(hex2dec('12')),wire_in_4,wire_in_4)\n        updatewireins(dev)\n        wire_in_5=fifo_th;\n        setwireinvalue(dev,int32(hex2dec('13')),wire_in_5,wire_in_5)\n        updatewireins(dev)\n        wire_in_6=offset_clk_cycles;\n        setwireinvalue(dev,int32(hex2dec('14')),wire_in_6,wire_in_6)\n        updatewireins(dev)\n\n        % BEGIN SAVE\n\n        rep_no=fix(no_gate_pos_m/buffer_frame_size);\n        [daq_time]=ss2_daq_hdf5_v3(file_name,rep_no,dev,int32(hex2dec('A0')),16384,(512*256)*buffer_frame_size);\n    \n        %%%%%%%%%%%%%%%%%%%%%%%%%%%%%%%%%%%%%%\n        % Added by XM for hdf5 saving purposes\n\n        disp(['Elapsed DAQ time: ' num2str(daq_time) ' sec']);\n\n        % end XM additions\n        %%%%%%%%%%%%%%%%%%%%%%%%%%%%%%%%%%%%%%\n\n%         updatewireouts(dev);\n%         fsm_state = dec2hex(getwireoutvalue(dev,int32(hex2dec('20'))));    \n        updatewireouts(dev);\n        fsm_state_2 = dec2hex(getwireoutvalue(dev,int32(hex2dec('21'))));\n\n        beep\n \n        disp([10 'ACQUISITION COMPLETED. YOU CAN TURN OFF THE LASER NOW.' 10])\n%         fsm_state_int=str2double(fsm_state_2);\n%         if fsm_state_int==2\n%             disp(['USB DATA TRANSFER SUCCESSFUL!' 10])\n%         else\n%             disp(['USB DATA TRANSFER FAILED!' 10])\n%         end\n        \n%         file_number_str=int2str(i);\n%         disp(['SAVING HDF5 RAW DATA... File ' file_number_str ' of ' repetition_number_str config_number_str 10])\n\n    end\nend\n\ncloseFPGA(dev);\n\nhdf5write([currentFolder '\\raw_data\\' file_name '.hdf5'],'/daq_time_s',daq_time,'WriteMode', 'append');\n\n% end XM additions\n%%%%%%%%%%%%%%%%%%%%%%%%%%%%%%%%%%%%%%\n    \n%% \n\n%%%%%%%%%%%%%%%%%%%%%%%%%%%%%%%%%%%%%%\n% Added by AU for testing purposes\n\n% disp([10 'SAVING .MAT RAW DATA...' 10])\n% \n% tic\n% \n% save([currentFolder '\\raw_data\\raw_data_1.mat'],'SS2_DATA', '-v7.3');\n% \n% toc\n\n% end AU additions\n%%%%%%%%%%%%%%%%%%%%%%%%%%%%%%%%%%%%%%\n\ndisp([10 'DONE.'])\n\n%disp('SAVING MATLAB RAW DATA...')\n\n%tic\n%save([currentFolder '\\raw_data\\' file_name '_' file_number_str '.mat'],'CC');\n%toc\n\nbeep"
      # "# images = # gates/set (8-bit)\nor 4 x # gates/set (10-bit)"
      # "buffer size = 1 (8-bit) or 4 (10-bit)"
      n16 = Unbundle By Name(w117) -> ("10 bits"=w112:bool, "Gate Offset"=w87:u32, "# Gates per Set"=w115:u32, "# Exposure Sequences"=w114:u32, "Gate Definition.gs_psincdec_0"=w102:u32, "Gate Definition.gs_psincdec_1"=w101:u32, "Gate Definition.gs_psincdec_2"=w100:u32, "Gate Definition.gs_psincdec_3"=w99:u32, "Gate Definition.gs_no_shift_adj_1"=w98:u32, "Gate Definition.gs_no_shift_adj_2"=w97:u32, "Gate Definition.gs_no_shift_adj_3"=w96:u32, "Gate Shift"=w110:u32, "# Sets"=w104:u32)
      n17 = case shown="False" w113 {
        tunnel: w112 -> [w133 _]
        tunnel: [w133 _] -> w111
        tunnel: w110 -> [w132 _]
        tunnel: [w132 _] -> w109
        tunnel: w104 -> [w131 _]
        tunnel: [w131 u32 1 ("# Sets")] -> w103
        tunnel: w102 -> [w130 _]
        tunnel: w101 -> [w129 _]
        tunnel: w100 -> [w128 _]
        tunnel: w99 -> [w127 _]
        tunnel: w98 -> [w126 _]
        tunnel: w97 -> [w125 _]
        tunnel: w96 -> [w124 _]
        tunnel: [w130 _] -> w95
        tunnel: [w129 _] -> w94
        tunnel: [w128 _] -> w93
        tunnel: [w127 _] -> w92
        tunnel: [w126 _] -> w91
        tunnel: [w125 _] -> w90
        tunnel: [w124 _] -> w89
        frame False {
          # "Recording"
        }
        frame True {
          # "Live Mode"
        }
      }
      n18 = Boolean To (0,1)(Boolean=w111) -> (0, 1=w116:i16)
      n19 = formula code="uInt32 no_gate_rep;\nuInt32 fifo_th,rows,no_gate_pos_m;\nuInt32 wire_in_0,wire_in_1,wire_in_2,wire_in_3,wire_in_4,wire_in_5,wire_in_6;\nfloat64 offset_time_seconds;\nuInt32 offset_clk_cycles, buffer_frame_size;\n\n// BEGIN user parameters\n\n// buffer_frame_size=40; % the size of the RAM buffer in terms of \n// equivalent 256*512 8-bit frames = 128 kB\n// choose a value that no_gate_pos is divisible by.\n\n// bits_10 = 0; % 1: 10-bit images, 0: 8-bit images\n// gate_offset = 2025; % number of gates to skip before data acquisition (default: 0): now defined as part of config_array\n// no_gate_pos = 1000; % number of gate positions per gate set\n// exp_no_seq = 25; % (exposure=400ns*exp_no_seq-50ns)\n// gs_no_shift = 1; % gate shift between 2 subsequent gate positions (x 17.857 ps)\n\n// gs_psincdec_0 = 1; % direction of the gate wrt the laser (0: backward, 1: forward)\n// gs_no_shift_adj_1 = 65; % gate window adjustment\n// gs_no_shift_adj_2 = 90; % gate window adjustment\n// gs_no_shift_adj_3 = 615; % gate window adjustment: now defined as part of config_array\n// gs_psincdec_1 = 0; % gate window adjustment\n// gs_psincdec_2 = 0; % gate window adjustment\n// gs_psincdec_3 = 1; % gate window adjustment: now defined as part of config_array\n\n// END user parameters\n\noffset_time_seconds=0.001; //min: 1E-6, max: 9\noffset_clk_cycles=floor(offset_time_seconds/(5E-9));\nno_gate_rep = 255; // number of bits in each gate position (this should remain 255)\nfifo_th=16384;\n//rows = 256;\n\n no_gate_pos_m = (bits_10 ==1) ? no_gate_pos*4 : no_gate_pos;\nbuffer_frame_size = (bits_10 ==1) ? 4 : 1;\n//was: = no_gate_pos_m; // e.g. bits_10 = 1, no_gate_pos = 100 >> buffer = 50 MB\n//no_gate_pos_m *= n_sets; \n//no_rows = rows-1;\n//frames=no_gate_rep;\n\n//wire_in_0=gs_psincdec_0+gs_psincdec_1*2**1+gs_psincdec_2*2**2+gs_psincdec_3*2**3+gs_no_shift_adj_1*2**4+bits_10*2**19;\nwire_in_0 = 0;\n//wire_in_1=gs_no_shift_adj_2+gs_no_shift_adj_3*2**15;\nwire_in_1 = 0;\n//wire_in_2=no_gate_pos_m*2**8;\nwire_in_2=2**8;\n//wire_in_3=exp_no_seq+gate_offset*2**16;\nwire_in_3 = exp_no_seq;\n//wire_in_4=gs_no_shift;\nwire_in_4 = 0;\nwire_in_5=fifo_th;\nwire_in_6=offset_clk_cycles;" "From sequential_data_v2_acq_AU_v3.m"("bits_10"=w116, "gate_offset"=w87, "no_gate_pos"=w115, "exp_no_seq"=w114, "gs_psincdec_0"=w95, "gs_psincdec_1"=w94, "gs_psincdec_2"=w93, "gs_psincdec_3"=w92, "gs_no_shift_adj_1"=w91, "gs_no_shift_adj_2"=w90, "gs_no_shift_adj_3"=w89, "gs_no_shift"=w109, "n_sets"=w103) -> ("wire_in_1"=w122:u32, "wire_in_0"=w123:u32, "wire_in_2"=w121:u32, "wire_in_3"=w120:u32, "no_gate_pos_m"=w105:u32, "wire_in_4"=w108:u32, "wire_in_5"=w107:u32, "wire_in_6"=w106:u32, "buffer_frame_size"=w88:u32)
      n20 = Build Array(w123, w122, w121, w120, w108, w107, w106) -> (w119:u32[])
    }
  }
  "SS2 FPGA DAQ Parameters" <- w14
  "Error Out" <- w6
  "SS2 FPGA DAQ Addresses" <- w13
  "#8-bit Images per Set" <- w10
  "Discard First Image" <- w2
  "Buffer Size (#8-bit Images)" <- w1
